vi "Gryo aline.vi"(8 "Joystick Control":dbl, 11 "Current Gyro Val":dbl) -> (1 "Output":dbl)   [LabVIEW 2014]
uses:
  <vilib>/addons/control/pid/pid.llb/PID (DBL).vi
  <vilib>/addons/control/pid/NI_PID_pid.lvlib
panel:
  out "Setpoint 2":dbl
  in  "Reset Setpoint":bool
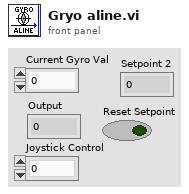
[diagram p1: front panel]
types:
  T1 = cluster{"proportional gain (Kc)":dbl, "integral time (Ti, min)":dbl, "derivative time (Td, min)":dbl}
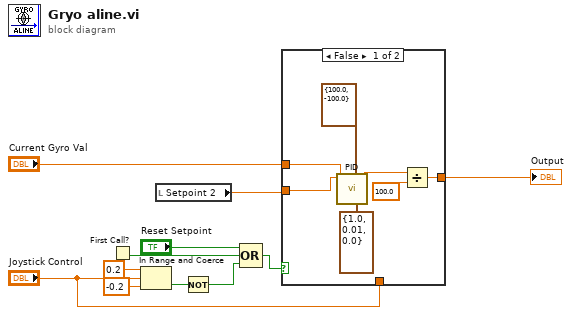
[diagram p0: block diagram]
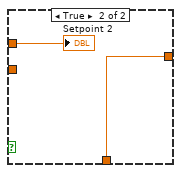
[diagram p2: hidden frame]
diagram:
  n1 = First Call?() -> (First Call?: T/F=w3:bool)
  n2 = In Range and Coerce(upper limit=0.2, x="Joystick Control", lower limit=-0.2 ("y")) -> (In Range?=w8:bool)  [unwired: 1 out]
  n3 = local read "Setpoint 2"() -> (w7:dbl)
  n4 = Not(x=w8) -> (.not. x?=w1:bool)
  n5 = Compound Arithmetic op=OR("Reset Setpoint", w3, w1) -> (w2:bool)
  n6 = case shown="False" w2 {
    tunnel: w7 -> [w12 _]
    tunnel: "Current Gyro Val" -> [w18 w19]
    tunnel: [w15 w20] -> w6
    tunnel: "Joystick Control" -> [_ w20]
    frame False {
      n7 = call-poly <vilib>:"PID.vi"("output range"=cluster{"output high":dbl, "output low":dbl} {"output high"=100.0, "output low"=-100.0}, "PID gains"=T1 {"proportional gain (Kc)"=1.0, "integral time (Ti, min)"=0.01, "derivative time (Td, min)"=0.0}, "process variable"=w18, "setpoint"=w12) -> ("output"=w14:dbl)  [unwired: 6 in, 1 out]
      n8 = Divide(x=w14, y=100.0) -> (x/y=w15:dbl)
    }
    frame True {
      "Setpoint 2" <- w19
    }
  }
  "Output" <- w6
